vi "On Compile - Parse System Definition and Initialize Data Refs.vi"(8 "error in":errorcluster, 11 "custom device ref in":T1 format="%.0x") -> (0 "error out":errorcluster)   [LabVIEW 2020, in "Communication Bus Template System Explorer.lvlib" / "Implementation.lvlib"]
uses:
  Implementation.lvlib
  <vilib>/NI VeriStand/Custom Device API/Custom Device Item Ref.ctl
  Shared/RT Hardware Channel Settings.ctl
  Shared/RT Label Settings.ctl
  Shared/Label.ctl
  Shared/RT Parameters.ctl
  Shared/Parameter Definition.ctl
  Encoding and Decoding/Encoding.ctl
  <vilib>/NI VeriStand/Custom Device API/Block Data Reference.ctl
  <vilib>/NI VeriStand/Custom Device API/Data Reference.ctl
  Shared/Transfer Type.ctl
  Scripting/Constants.vi
  <vilib>/NI VeriStand/Custom Device API/Set Item Property (Variant).vi
  <vilib>/NI VeriStand/Custom Device API/Custom Device API.lvlib
  Encoding and Decoding/Encoding and Decoding.lvlib
  Scripting/Communication Bus Template Scripting.lvlib
  <vilib>/NI/NIVS Inline Async API/_Data Access System Explorer/Data Access System Explorer.lvlib
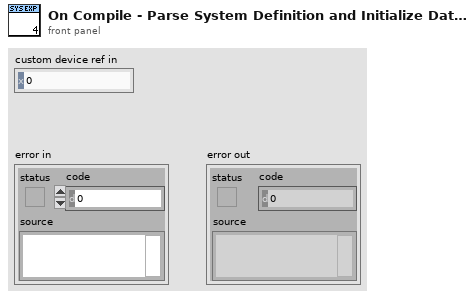
[diagram p1: front panel]
types:
  T1 = typedef "Custom Device API.lvlib/Custom Device Item Ref.ctl" = u64
  T2 = typedef "RT Hardware Channel Settings.ctl" = cluster{"channel #":u16, "channel handle":u64, "labels settings for RT":T3[]}
  T3 = typedef "RT Label Settings.ctl" = cluster{"Name":string, "xmlName":string, "label":T4, "transfer period":u32, "SDI_Enabled":bool, "SDI":u8, "parameter driver data":T5, "transfer type":T10, "has timestamp?":bool, "Label Disable/Trigger Channel Reference":T1, "Message Handle":u64, "Initialized?":bool, "Word Initial Raw Value":u32, "Label Timestamp Channel Data Reference":T9}
  T4 = typedef "Label.ctl" = u8
  T5 = typedef "RT Parameters.ctl" = cluster{"parameter definitions":T6[], "Rx block data refs":T8[], "Rx values":dbl[], "Tx parameter refs":T1[]}
  T6 = typedef "Parameter Definition.ctl" = cluster{"start index":i32, "size":i32, "encoding":T7, "signed":bool, "scale multiplier":dbl, "scale offset":dbl}
  T7 = typedef "Encoding and Decoding.lvlib/Encoding.ctl" = enum16{"BNR", "BCD", "Discrete"}
  T8 = typedef "Custom Device API.lvlib/Block Data Reference.ctl" = cluster{"Data Reference":T9, "Offset":u64, "Length":u64}
  T9 = typedef "Custom Device API.lvlib/Data Reference.ctl" = i32
  T10 = typedef "Transfer Type.ctl" = enum16{"Scheduled", "Acyclic", "Block", "Strobe"}
  T11 = cluster{"Name":string, "Rx configuration":T2[], "Tx configuration":T2[]}
  T12 = typedef "Custom Device API.lvlib/Custom Device Item Info.ctl" = cluster{"Name":string, "Is Channel":bool, "GUID":string, "Is Waveform":bool}
  T13 = cluster{"Name":string, "Type":enum16{"Output/Write", "Input/Read", "Input/ReadWrite"}, "VS Refs":T1[]}
  T14 = cluster{"Name":string, "Type":enum16{"Output/Write", "Input/Read", "Input/ReadWrite"}, "VS Refs":T1[]}[]
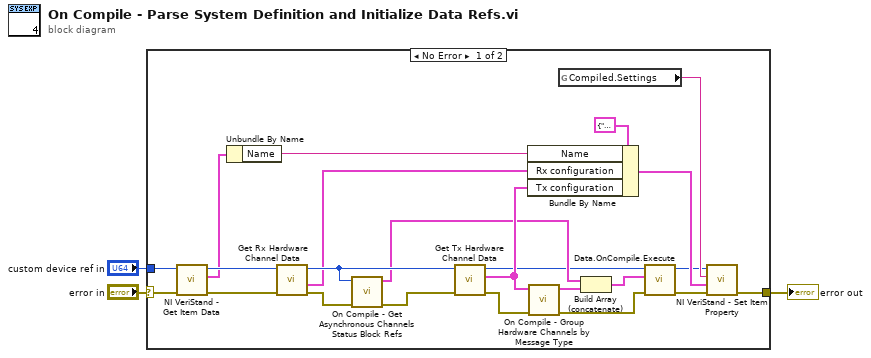
[diagram p0: block diagram]
diagram:
  n1 = case shown="No Error" "error in" {
    selector: "error in" -> [w16 w27]
    tunnel: "custom device ref in" -> [w26 _]
    tunnel: [w15 w27] -> w1
    frame No Error {
      n2 = call <vilib>:"NI VeriStand - Get Item Data.vi"("error in (no error)"=w16, "Item Ref in"=w26) -> ("error out"=w24:errorcluster, "Item Info"=w23:T12, "Item Ref out"=w25:T1)  [unwired: 6 in, 1 out]
      n3 = Unbundle By Name(w23) -> ("Name"=w22:string)
      n4 = call "Get Rx Hardware Channel Data.vi"("error in"=w24, "custom device ref in"=w25) -> ("error out"=w13:errorcluster, "Rx hardware channel data"=w4:T2[], "custom device ref out"=w14:T1)  [unwired: 6 in, 1 out]
      n5 = call "On Compile - Get Asynchronous Channels Status Block Refs.vi"("error in"=w13, "Item Ref"=w14) -> ("error out"=w12:errorcluster, "Async Status Channels Refs"=w6:T13)  [unwired: 8 in]
      n6 = call "Get Tx Hardware Channel Data.vi"("error in"=w12, "custom device ref in"=w14) -> ("error out"=w8:errorcluster, "Tx hardware channel data"=w10:T2[], "custom device ref out"=w5:T1)  [unwired: 7 in]
      n7 = Bundle By Name(cluster=T11 {"Name"="", "Rx configuration"=[], "Tx configuration"=[]}, "Name"=w22, "Rx configuration"=w4, "Tx configuration"=w10) -> (w19:T11)
      n8 = call "On Compile - Group Hardware Channels by Message Type.vi"("error in"=w8, "hardware channel data"=w10) -> ("error out"=w7:errorcluster, "grouped hardware channel data refs"=w9:T14)  [unwired: 8 in]
      n9 = global read "Constants.vi" "Compiled.Settings"() -> (w20:string)
      n10 = Build Array (concatenate)(w6, w9) -> (w11:T14)
      n11 = call <vilib>:"Data.OnCompile.Execute.vi"("error in"=w7, "VS Ref Groups"=w11, "Custom Device Ref"=w5) -> ("error out"=w17:errorcluster, "Custom Device Ref"=w18:T1)  [unwired: 7 in]
      n12 = call-poly <vilib>:"NI VeriStand - Set Item Property.vi"("error in (no error)"=w17, "Value"=w19, "Property Name"=w20, "Item Ref in"=w18) -> ("error out"=w15:errorcluster)  [unwired: 5 in, 2 out]
    }
    frame Error {
    }
  }
  "error out" <- w1
